vi "BAE4.vi"() -> ()   [LabVIEW 2014]
doc: "BAE4\n\nDisplays a graph of of phi and theta angles from the time and position difference from three sensor positions and the origin. It also checks the validity of the source.\n\nSubvis used: build event cluster start, calculate polat angles for unit vector, calculate unit vector component, conv from ns to time clust, convert from time clust to ns, distribution generator, event data analysis start, generate polar angle distribution, generate time clusters\n\nBeverly Abadines\nPHY 350\nE4"
uses:
  typedefs/unit vector typedef.ctl
  typedefs/event cluster typedef.ctl
  typedefs/positions cluster typedef.ctl
  typedefs/time cluster typedef.ctl
  typedefs/polar angle typedef.ctl
panel:
  out "polar plot":cluster{sgl[], sgl[]}(graph)
  out "polar angles to mean":T1={"theta [degrees]"=115.59249, "phi [degrees]"=-131.44662}
  in  "c [m/s]":sgl=300000000.0 caption="speed of light [m/s]"
  in  "sensor positions":T2(tab)
  out "origin times":T3[](array[typedef])=[{"day"=1, "hour"=5, "min"=11, "sec"=27, "msec"=34, "usec"=310, "nsec"=314}, {"day"=1, "hour"=5, "min"=11, "sec"=27, "msec"=34, "usec"=240, "nsec"=513}, {"day"=1, "hour"=5, "min"=11, "sec"=27, "msec"=33, "usec"=753, "nsec"=636}, {"day"=1, "hour"=5, "min"=11, "sec"=27, "msec"=33, "usec"=933, "nsec"=585}, {"day"=1, "hour"=5, "min"=11, "sec"=27, "msec"=34, "usec"=243, "nsec"=307}, {"day"=1, "hour"=5, "min"=11, "sec"=27, "msec"=33, "usec"=952, "nsec"=670}]
  out "deviation from mean origin":T4(graph)={"X Values"=[-290867.6, -235199.8, -179532.0, -123864.2, -68196.4, -12528.6, 43139.2, 98807.0, 154474.8, 210142.6], "Histogram: h(x)"=[1, 0, 0, 2, 0, 0, 0, 0, 2, 1]}
  out "events origin":T5[](array[typedef])=[{"position [km]"=0.0, "time [nsec]"=105087034310314}, {"position [km]"=0.0, "time [nsec]"=105087034240513}, {"position [km]"=0.0, "time [nsec]"=105087033753636}, {"position [km]"=0.0, "time [nsec]"=105087033933585}, {"position [km]"=0.0, "time [nsec]"=105087034243307}, {"position [km]"=0.0, "time [nsec]"=105087033952670}]
  out "average event origin":T5={"position [km]"=0.0, "time [nsec]"=105087034072338}
  out "standard deviation orgin (ns)":i32=51641
  out "number of events origin":i32=14
  out "average event a":T5={"position [km]"=0.0, "time [nsec]"=105087034072338}
  out "events a":T5[](array[typedef])=[{"position [km]"=0.0, "time [nsec]"=105087034310314}, {"position [km]"=0.0, "time [nsec]"=105087034240513}, {"position [km]"=0.0, "time [nsec]"=105087033753636}, {"position [km]"=0.0, "time [nsec]"=105087033933585}, {"position [km]"=0.0, "time [nsec]"=105087034243307}, {"position [km]"=0.0, "time [nsec]"=105087033952670}]
  out "number of events a":i32=6
  out "standard deviation a (ns)":i32=223289
  out "deviation from mean a":T4(graph)={"X Values"=[-290867.6, -235199.8, -179532.0, -123864.2, -68196.4, -12528.6, 43139.2, 98807.0, 154474.8, 210142.6], "Histogram: h(x)"=[1, 0, 0, 2, 0, 0, 0, 0, 2, 1]}
  out "a times":T3[](array[typedef])=[{"day"=1, "hour"=5, "min"=11, "sec"=27, "msec"=37, "usec"=85, "nsec"=571}, {"day"=1, "hour"=5, "min"=11, "sec"=27, "msec"=37, "usec"=177, "nsec"=518}, {"day"=1, "hour"=5, "min"=11, "sec"=27, "msec"=36, "usec"=988, "nsec"=557}, {"day"=1, "hour"=5, "min"=11, "sec"=27, "msec"=37, "usec"=107, "nsec"=406}, {"day"=1, "hour"=5, "min"=11, "sec"=27, "msec"=37, "usec"=108, "nsec"=720}, {"day"=1, "hour"=5, "min"=11, "sec"=27, "msec"=37, "usec"=269, "nsec"=604}, {"day"=1, "hour"=5, "min"=11, "sec"=27, "msec"=37, "usec"=149, "nsec"=158}, {"day"=1, "hour"=5, "min"=11, "sec"=27, "msec"=37, "usec"=85, "nsec"=989}, {"day"=1, "hour"=5, "min"=11, "sec"=27, "msec"=37, "usec"=153, "nsec"=696}, {"day"=1, "hour"=5, "min"=11, "sec"=27, "msec"=37, "usec"=126, "nsec"=156}]
  out "average event b":T5={"position [km]"=0.0, "time [nsec]"=105087034072338}
  out "events b":T5[](array[typedef])=[{"position [km]"=0.0, "time [nsec]"=105087034310314}, {"position [km]"=0.0, "time [nsec]"=105087034240513}, {"position [km]"=0.0, "time [nsec]"=105087033753636}, {"position [km]"=0.0, "time [nsec]"=105087033933585}, {"position [km]"=0.0, "time [nsec]"=105087034243307}, {"position [km]"=0.0, "time [nsec]"=105087033952670}]
  out "number of events b":i32=6
  out "deviation from mean b":T4(graph)={"X Values"=[-290867.6, -235199.8, -179532.0, -123864.2, -68196.4, -12528.6, 43139.2, 98807.0, 154474.8, 210142.6], "Histogram: h(x)"=[1, 0, 0, 2, 0, 0, 0, 0, 2, 1]}
  out "standard deviation b (ns)":i32=223289
  out "b times":T3[](array[typedef])=[{"day"=1, "hour"=5, "min"=11, "sec"=27, "msec"=36, "usec"=825, "nsec"=132}, {"day"=1, "hour"=5, "min"=11, "sec"=27, "msec"=36, "usec"=885, "nsec"=819}, {"day"=1, "hour"=5, "min"=11, "sec"=27, "msec"=36, "usec"=803, "nsec"=659}, {"day"=1, "hour"=5, "min"=11, "sec"=27, "msec"=36, "usec"=856, "nsec"=103}, {"day"=1, "hour"=5, "min"=11, "sec"=27, "msec"=36, "usec"=852, "nsec"=907}, {"day"=1, "hour"=5, "min"=11, "sec"=27, "msec"=36, "usec"=846, "nsec"=163}, {"day"=1, "hour"=5, "min"=11, "sec"=27, "msec"=36, "usec"=814, "nsec"=697}, {"day"=1, "hour"=5, "min"=11, "sec"=27, "msec"=36, "usec"=799, "nsec"=794}, {"day"=1, "hour"=5, "min"=11, "sec"=27, "msec"=36, "usec"=833, "nsec"=769}, {"day"=1, "hour"=5, "min"=11, "sec"=27, "msec"=36, "usec"=752, "nsec"=951}, {"day"=1, "hour"=5, "min"=11, "sec"=27, "msec"=36, "usec"=822, "nsec"=343}, {"day"=1, "hour"=5, "min"=11, "sec"=27, "msec"=36, "usec"=866, "nsec"=81}, {"day"=1, "hour"=5, "min"=11, "sec"=27, "msec"=36, "usec"=821, "nsec"=612}, {"day"=1, "hour"=5, "min"=11, "sec"=27, "msec"=36, "usec"=777, "nsec"=584}, {"day"=1, "hour"=5, "min"=11, "sec"=27, "msec"=36, "usec"=791, "nsec"=505}, {"day"=1, "hour"=5, "min"=11, "sec"=27, "msec"=36, "usec"=867, "nsec"=724}, {"day"=1, "hour"=5, "min"=11, "sec"=27, "msec"=36, "usec"=761, "nsec"=271}]
  out "average event c":T5={"position [km]"=0.0, "time [nsec]"=105087034072338}
  out "events c":T5[](array[typedef])=[{"position [km]"=0.0, "time [nsec]"=105087034310314}, {"position [km]"=0.0, "time [nsec]"=105087034240513}, {"position [km]"=0.0, "time [nsec]"=105087033753636}, {"position [km]"=0.0, "time [nsec]"=105087033933585}, {"position [km]"=0.0, "time [nsec]"=105087034243307}, {"position [km]"=0.0, "time [nsec]"=105087033952670}]
  out "number of events c":i32=6
  out "deviation from mean c":T4(graph)={"X Values"=[-290867.6, -235199.8, -179532.0, -123864.2, -68196.4, -12528.6, 43139.2, 98807.0, 154474.8, 210142.6], "Histogram: h(x)"=[1, 0, 0, 2, 0, 0, 0, 0, 2, 1]}
  out "standard deviation c (ns)":i32=223289
  out "c times":T3[](array[typedef])=[{"day"=1, "hour"=5, "min"=11, "sec"=27, "msec"=35, "usec"=596, "nsec"=675}, {"day"=1, "hour"=5, "min"=11, "sec"=27, "msec"=35, "usec"=625, "nsec"=654}, {"day"=1, "hour"=5, "min"=11, "sec"=27, "msec"=35, "usec"=624, "nsec"=427}, {"day"=1, "hour"=5, "min"=11, "sec"=27, "msec"=35, "usec"=652, "nsec"=689}, {"day"=1, "hour"=5, "min"=11, "sec"=27, "msec"=35, "usec"=611, "nsec"=295}, {"day"=1, "hour"=5, "min"=11, "sec"=27, "msec"=35, "usec"=622, "nsec"=850}]
  in  "positions":T6={"a [km]"=1535.0, "b [km]"=1221.0, "c [km]"=1077.0} caption="positions [km]"
  out "unit vector to mean":T7={"nx"=-0.596658, "ny"=-0.6756666, "nz"=-0.43173456}
  out "checksum":sgl=0.9994603
  out "signal valid":bool=TRUE
  # "Beverly Abadines\nPHY 350\nE4"
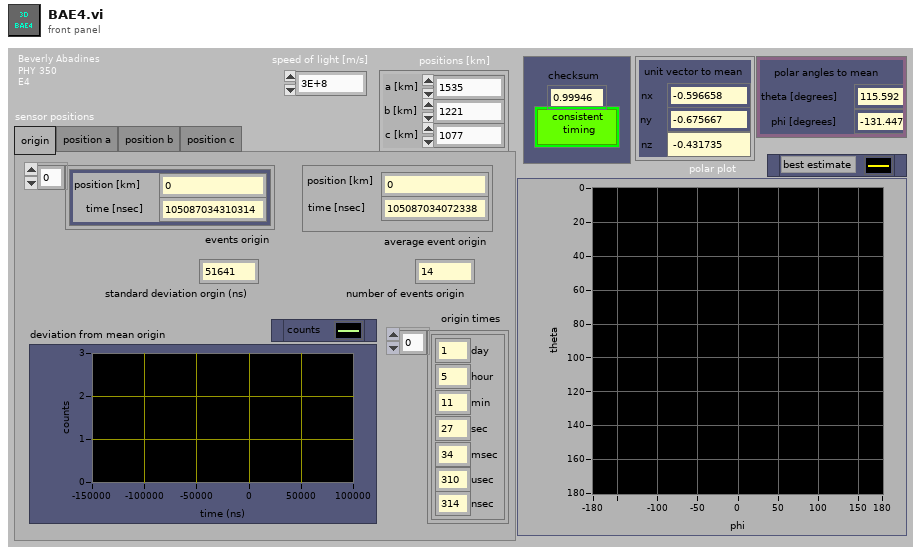
[diagram p1: front panel]
types:
  T1 = typedef "polar angle typedef.ctl" = cluster{"theta [degrees]":sgl, "phi [degrees]":sgl}
  T2 = enum32{"origin", "position a", "position b", "position c"}
  T3 = typedef "time cluster typedef.ctl" = cluster{"day":u32, "hour":u32, "min":u32, "sec":u32, "msec":u32, "usec":u32, "nsec":u32}
  T4 = cluster{"X Values":dbl[], "Histogram: h(x)":i32[]}
  T5 = typedef "event cluster typedef.ctl" = cluster{"position [km]":sgl, "time [nsec]":i64}
  T6 = typedef "positions cluster typedef.ctl" = cluster{"a [km]":sgl, "b [km]":sgl, "c [km]":sgl}
  T7 = typedef "unit vector typedef.ctl" = cluster{"nx":sgl, "ny":sgl, "nz":sgl}
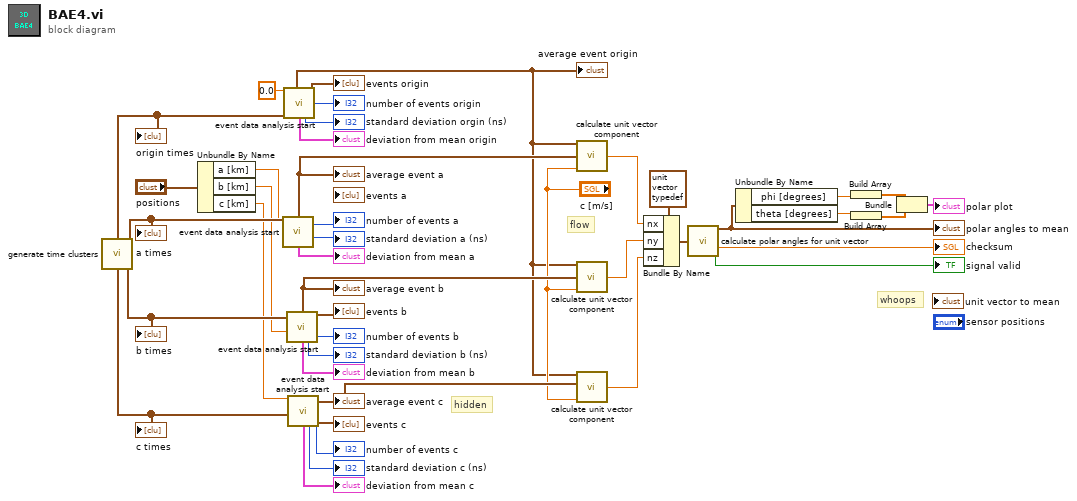
[diagram p0: block diagram]
diagram:
  # "hidden"
  # "whoops"
  # "flow"
  n1 = call "generate time clusters.vi"() -> ("origin times"=w42:T3[], "position a times"=w37:T3[], "position c times"=w24:T3[], "position b times"=w25:T3[])  [unwired: 12 in]
  "origin times" <- w42
  "a times" <- w37
  "b times" <- w25
  "c times" <- w24
  n2 = Unbundle By Name("positions") -> ("a [km]"=w22:sgl, "b [km]"=w21:sgl, "c [km]"=w20:sgl)
  n3 = call "event data analysis start.vi"("position in [km]"=w22, "times in"=w37) -> ("average event"=w19:T5, "num of events"=→"number of events a":i32, "histogram"=→"deviation from mean a":T4, "standard deviation (ns)"=→"standard deviation a (ns)":i32)  [unwired: 8 in, 2 out]
  "average event a" <- w19
  n4 = call "event data analysis start.vi"("position in [km]"=sgl 0.0, "times in"=w42) -> ("average event"=w7:T5, "events"=→"events origin":T5[], "num of events"=→"number of events origin":i32, "histogram"=→"deviation from mean origin":T4, "standard deviation (ns)"=→"standard deviation orgin (ns)":i32)  [unwired: 8 in, 1 out]
  "average event origin" <- w7
  n5 = call "event data analysis start.vi"("position in [km]"=w21, "times in"=w25) -> ("average event"=w17:T5, "events"=→"events b":T5[], "num of events"=→"number of events b":i32, "histogram"=→"deviation from mean b":T4, "standard deviation (ns)"=→"standard deviation b (ns)":i32)  [unwired: 8 in, 1 out]
  "average event b" <- w17
  n6 = call "event data analysis start.vi"("position in [km]"=w20, "times in"=w24) -> ("average event"=w16:T5, "events"=→"events c":T5[], "num of events"=→"number of events c":i32, "histogram"=→"deviation from mean c":T4, "standard deviation (ns)"=→"standard deviation c (ns)":i32)  [unwired: 8 in, 1 out]
  "average event c" <- w16
  n7 = call "calculate unit vector component.vi"("event data at origin in"=w7, "event data along axis in"=w19, "speed of light [m/s]"="c [m/s]") -> ("component of unit vector"=w18:sgl)  [unwired: 12 in]
  n8 = call "calculate unit vector component.vi"("event data at origin in"=w7, "event data along axis in"=w17, "speed of light [m/s]"="c [m/s]") -> ("component of unit vector"=w14:sgl)  [unwired: 12 in]
  n9 = call "calculate unit vector component.vi"("event data at origin in"=w7, "event data along axis in"=w16, "speed of light [m/s]"="c [m/s]") -> ("component of unit vector"=w13:sgl)  [unwired: 12 in]
  n10 = Bundle By Name(cluster=T7 {"nx"=-0.596658, "ny"=-0.6756666, "nz"=-0.43173456} ("unit vector to mean"), "nx"=w18, "ny"=w14, "nz"=w13) -> (w10:T7)
  n11 = call "calculate polar angles for unit vector.vi"("unit vector in"=w10) -> ("polar angles out"=w6:T1, "checksum"=→"checksum":sgl, "signal valid"=→"signal valid":bool)  [unwired: 12 in]
  "polar angles to mean" <- w6
  n12 = Unbundle By Name(w6) -> ("phi [degrees]"=w3:sgl, "theta [degrees]"=w4:sgl)
  n13 = Build Array(w3) -> (w2:sgl[])
  n14 = Build Array(w4) -> (w1:sgl[])
  n15 = Bundle(w2, w1) -> (→"polar plot":cluster{sgl[], sgl[]})  [unwired: 1 in]
